vi "GetNanonisScanPoint.vi"(6 "Internal use":string, 7 "Grid param":T1 {"height (m)" format="%#_6p"; "width (m)" format="%#_6p"; "center Y (m)" format="%#_6p"; "center X (m)" format="%#_6p"}, 8 "Error in (no error)":errorcluster, 9 "Points Y/Index Y":i32, 10 "Points X/Index X":i32, 11 "Method":enum16{"init", "run", "end"}(ring)) -> (0 "Error out":errorcluster)   [LabVIEW 2018]
doc: "Example of a measurement VI to be used in the \"Experiments on a Grid\" tool as external VI.\n\nThis example measures a potential difference map by performing bias spectroscopy and fitting a parabola to the Frequency Shift.\n\n- Nanonis Programming Interface -"
uses:
  <userlib>/Nanonis Prog Interface/Nanonis Prog Interface.lvlib
panel:
  in  "milliseconds to wait":u32
  # "\"Experiments on a Grid\" will first (before starting the measurements) call the external VI with the \"init\" method, passing the grid resolution (Points X, Points Y) and the grid dimensions (Grid param).\nThen, for the measurements, the external VI will be called with the \"run\" method, passing the current X and Y indices (Index X, Index Y).\nAfter the last measurement, the external VI will be called with the \"end\" method."
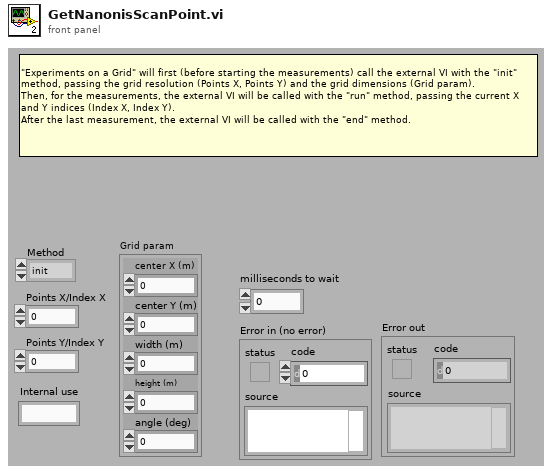
[diagram p1: front panel]
types:
  T1 = cluster{"center X (m)":sgl, "center Y (m)":sgl, "width (m)":sgl, "height (m)":sgl, "angle (deg)":sgl}
  T2 = enum16{"open", "replace", "create", "open or create", "replace or create", "replace or create with confirmation"}
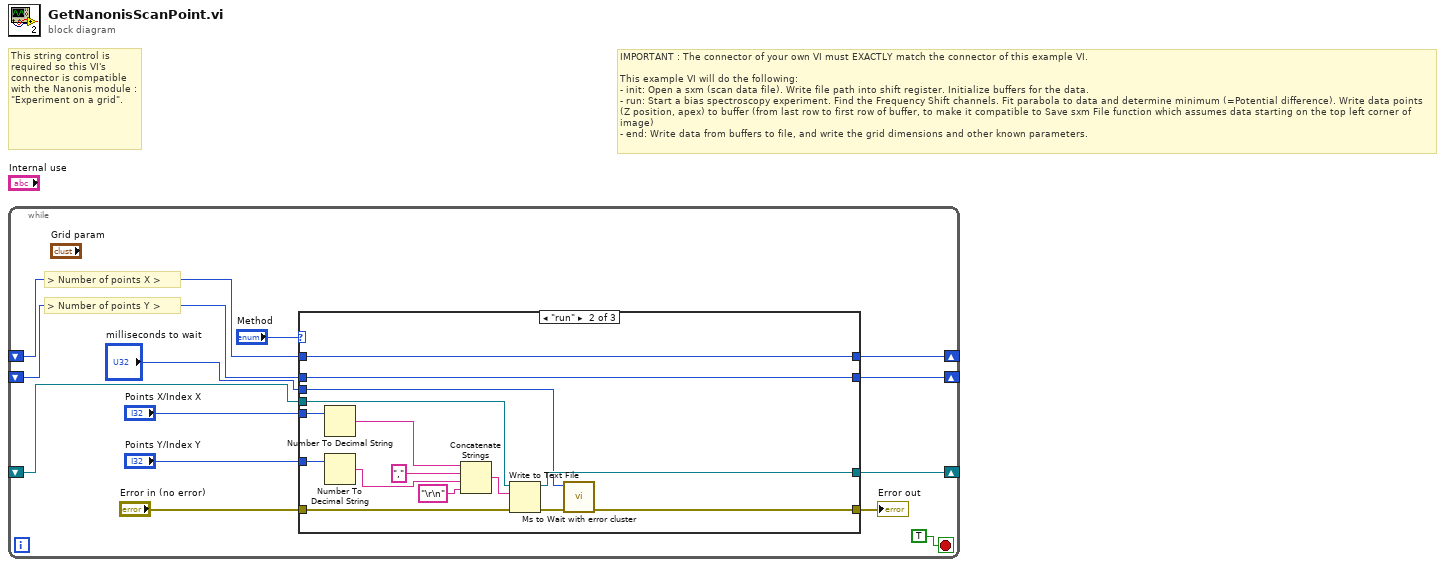
[diagram p0: block diagram]
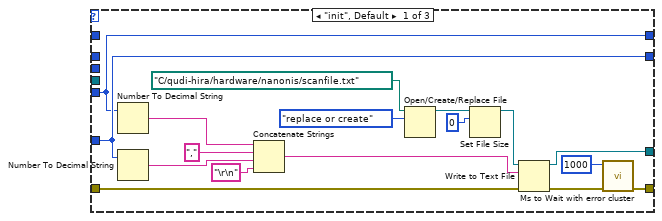
[diagram p2: hidden frame]
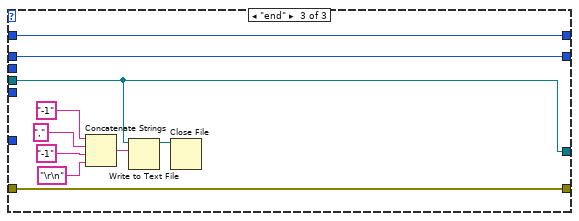
[diagram p3: hidden frame]
diagram:
  # "This string control is required so this VI's connector is compatible with the Nanonis module : \"Experiment on a grid\"."
  # "IMPORTANT : The connector of your own VI must EXACTLY match the connector of this example VI.\n\nThis example VI will do the following:\n- init: Open a sxm (scan data file). Write file path into shift register. Initialize buffers for the data.\n- run: Start a bias spectroscopy experiment. Find the Frequency Shift channels. Fit parabola to data and determine minimum (=Potential difference). Write data points (Z position, apex) to buffer (from last row to first row of buffer, to make it compatible to Save sxm File function which assumes data starting on the top left corner of image)\n- end: Write data from buffers to file, and write the grid dimensions and other known parameters."
  n1 = while {
    shift-right: [w8] -> _
    shift-left: _ -> [w7]
    shift-right: [w6] -> _
    shift-left: _ -> [w3]
    shift-right: [w5] -> _
    shift-left: _ -> [w4]
    stop <- TRUE stop-if-true
    # "> Number of points Y >"
    # "> Number of points X >"
    n2 = case shown="\"run\"" "Method" {
      tunnel: "Error in (no error)" -> [w15 w33 w46]
      tunnel: "Points X/Index X" -> [w18 w39 _]
      tunnel: "Points Y/Index Y" -> [w19 w38 _]
      tunnel: [w18 w44 w55] -> w8
      tunnel: w7 -> [_ w44 w55]
      tunnel: [w19 w45 w54] -> w6
      tunnel: w3 -> [_ w45 w54]
      tunnel: [w25 w36 w51] -> w5
      tunnel: w4 -> [_ w37 w51]
      tunnel: [w17 w31 w46] -> w2
      tunnel: "milliseconds to wait" -> [_ w34 _]
      frame "init", Default {
        n3 = Number To Decimal String(number=w18) -> (decimal integer string=w28:string)  [unwired: 1 in]
        n4 = Number To Decimal String(number=w19) -> (decimal integer string=w29:string)  [unwired: 1 in]
        n5 = Concatenate Strings(w28, "," ("string"), w29, "\r\n" ("string")) -> (w26:string)
        n6 = Open/Create/Replace File(file path (use dialog)=path "C:/qudi-hira/hardware/nanonis/scanfile.txt" ("Path"), operation (0:open)=T2."replace or create") -> (refnum out=w24:refnum<file>)  [unwired: 4 in, 2 out]
        n7 = Set File Size(6:i64 0 ("size (in bytes)"), 7:w24) -> (3:w23:refnum<file>)  [unwired: 1 in, 1 out]
        n8 = Write to Text File(file (use dialog)=w23, text=w26, error in=w15) -> (refnum out=w25:refnum<file>, error out=w14:errorcluster)  [unwired: 1 in, 1 out]
        n9 = call <userlib>:"Ms to Wait with error cluster.vi"("error in (no error)"=w14, "milliseconds to wait"=1000) -> ("error out"=w17:errorcluster)  [unwired: 4 in, 1 out]
      }
      frame "run" {
        n10 = Number To Decimal String(number=w39) -> (decimal integer string=w42:string)  [unwired: 1 in]
        n11 = Number To Decimal String(number=w38) -> (decimal integer string=w43:string)  [unwired: 1 in]
        n12 = Concatenate Strings(w42, "," ("string"), w43, "\r\n" ("string")) -> (w40:string)
        n13 = Write to Text File(file (use dialog)=w37, text=w40, error in=w33) -> (refnum out=w36:refnum<file>, error out=w32:errorcluster)  [unwired: 1 in, 1 out]
        n14 = call <userlib>:"Ms to Wait with error cluster.vi"("error in (no error)"=w32, "milliseconds to wait"=w34) -> ("error out"=w31:errorcluster)  [unwired: 4 in, 1 out]
      }
      frame "end" {
        n15 = Concatenate Strings("-1" ("string"), "," ("string"), "-1" ("string"), "\r\n" ("string")) -> (w52:string)
        n16 = Write to Text File(file (use dialog)=w51, text=w52) -> (refnum out=w50:refnum<file>)  [unwired: 2 in, 2 out]
        n17 = Close File(refnum=w50) -> ()  [unwired: 1 in, 2 out]
      }
    }
    "Error out" <- w2
  }
